vi "Delay in ms.vi"(8 "error in (no error)":errorcluster caption="Fehler (Eingang, kein Fehler)", 10 "Delay Time [ms]":u32) -> (0 "error out":errorcluster caption="Fehler (Ausgang)")   [LabVIEW 2017]
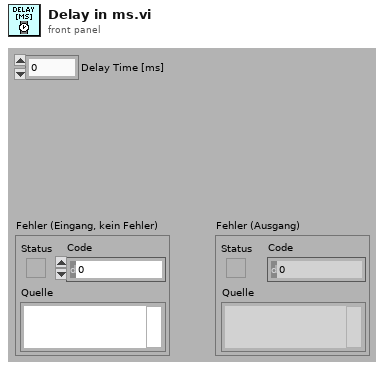
[diagram p1: front panel]
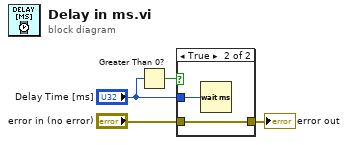
[diagram p0: block diagram]
diagram:
  n1 = Greater Than 0?(x="Delay Time [ms]") -> (x > 0?=w4:bool)
  n2 = case shown="True" w4 {
    tunnel: "Delay Time [ms]" -> [_ w7]
    tunnel: "error in (no error)" -> [w5 w6]
    tunnel: [w5 w6] -> w1
    frame False {
    }
    frame True {
      n3 = Wait (ms)(milliseconds to wait=w7) -> ()  [unwired: 1 out]
    }
  }
  "error out" <- w1
